vi "Unflatten JSONpath Array to Object.vi"(8 "error in (no error)":errorcluster, 9 "JSON Items":string[](array[string]), 11 "$Paths":string[](array[string])) -> (0 "error out":errorcluster, 3 "<JSON>":string)   [LabVIEW 2017, in "JSONtext.lvlib"]
doc: "Takes arrays of $Paths items and generates a Object containing those $Paths. Does not support multi-point paths.\n\nFor example: the $Paths (Items):\n$.A.B1 (1)\n$.A.B2 (\"x\")\n$.A2 (true)\n$.A3.C (123)\nproduce the JSON: {\"A\":{\"B1\":1\"B2:\"x\"},\"A2\":true,\"A3\":{\"C\":123}}"
uses:
  JSONtext.lvlib
  Parsing/Replace at Offset.vi
  support/Trim Input JSON (and null).vi
  Parsing/Advance past whitespace.vi
  <vilib>/JDP Science/JDP Science Common Utilities/Trim Whitespace__JDP.vi
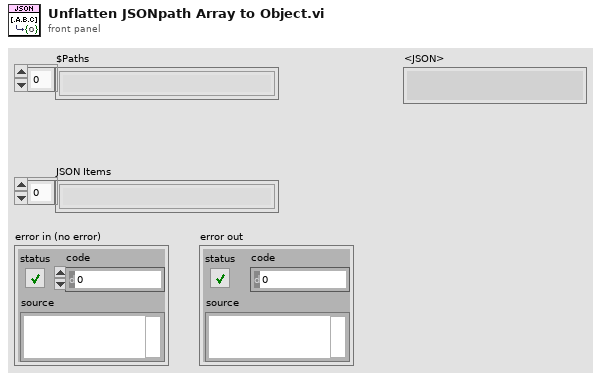
[diagram p1: front panel]
types:
  T1 = typedef "JSONtext.lvlib/Found Items.ctl" = cluster{"Item offset":i32, "Offset past Item":i32, "Name offset":i32, "Offset past Name":i32, "Found":bool, "Item Type":T2, "Item Index":i32}
  T2 = typedef "JSONtext.lvlib/Parsing State.ctl" = enum16{"Parser Error", "Object", "Array", "String", "Number/Other", "Leading Whitespace", "Object end", "Array end", "Value end"}
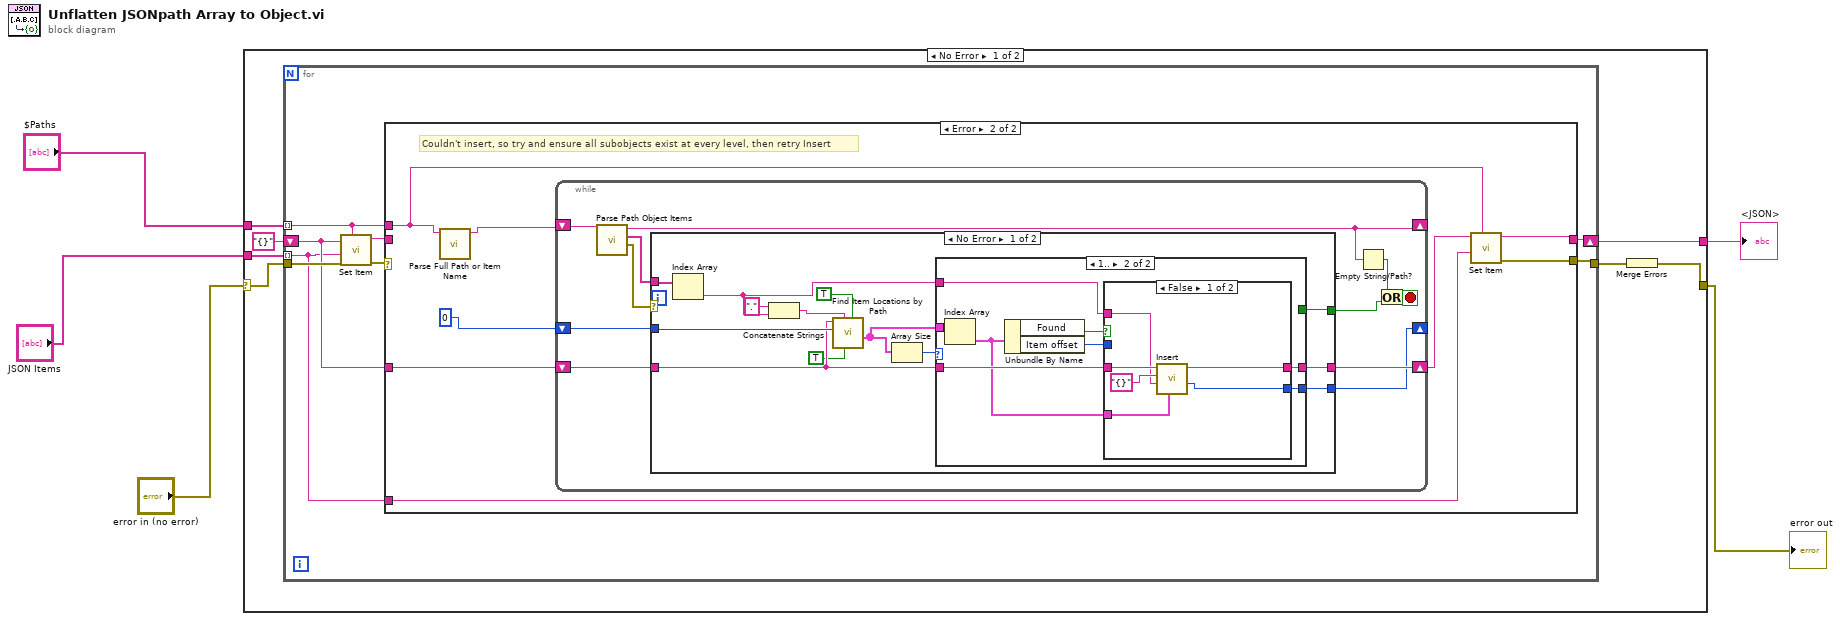
[diagram p0: block diagram]
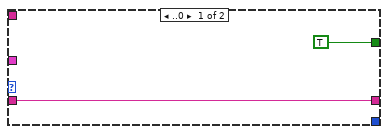
[diagram p3: hidden frame]
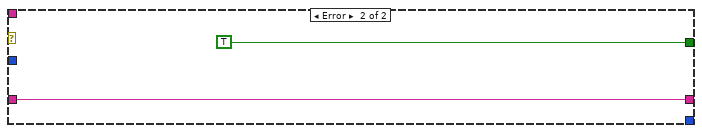
[diagram p5: hidden frame]
diagram:
  n1 = case shown="No Error" "error in (no error)" {
    selector: "error in (no error)" -> [w9 w75]
    tunnel: "$Paths" -> [w12 _]
    tunnel: "JSON Items" -> [w10 _]
    tunnel: [w8 _] -> w4
    tunnel: [w6 w75] -> w5
    frame No Error {
      n2 = for {
        tunnel: w12 -> [w18] mode=indexing
        shift-right: [w15] -> w8
        shift-left: "{}" ("<JSON>") -> [w17]
        tunnel: w10 -> [w13] mode=indexing
        tunnel: w9 -> [w20]
        tunnel: [w14] -> w7
        n3 = call "Set Item.vi"("$Path or Item Name"=w18, "error in (no error)"=w20, "JSON to Insert"=w13, "JSON"=w17) -> ("error out"=w19:errorcluster, "<JSON>"=w16:string)  [unwired: 4 in, 1 out]
        n4 = case shown="Error" w19 {
          selector: w19 -> [w21 _]
          tunnel: w18 -> [_ w25]
          tunnel: w17 -> [_ w30]
          tunnel: w16 -> [w22 _]
          tunnel: [w22 w28] -> w15
          tunnel: [w21 w27] -> w14
          tunnel: w13 -> [_ w26]
          frame No Error {
          }
          frame Error {
            # "Couldn't insert, so try and ensure all subobjects exist at every level, then retry Insert"
            n5 = call "Parse Full Path or Item Name.vi"("Full Path (with $) or Name"=w25) -> ("Relative Path or JSON-format name"=w23:string)  [unwired: 10 in]
            n6 = while {
              shift-right: [w39] -> _
              shift-left: w23 -> [w33]
              shift-right: [w36] -> w29
              shift-left: w30 -> [w37]
              shift-right: [w31] -> _
              shift-left: 0 ("Offset") -> [w32]
              stop <- w35 stop-if-true
              n7 = call "Parse Path Object Items.vi"("Path with leading Object element"=w33) -> ("error out"=w40:errorcluster, "<JSON>items names"=w38:string[], "Rest or Path"=w39:string)  [unwired: 8 in]
              n8 = case shown="No Error" w40 {
                tunnel: w38 -> [w54 _]
                tunnel: w37 -> [w51 w73]
                tunnel: [w53 w73] -> w36
                tunnel: [w43 TRUE] -> w34
                tunnel: w32 -> [w52 _]
                tunnel: [w48 _] -> w31
                frame No Error {
                  n9 = Index Array(array=w54) -> (element=w46:string)  [unwired: 1 in]
                  n10 = Concatenate Strings("." ("string"), w46) -> (w47:string)
                  n11 = call "Find Item Locations by Path.vi"("Insertion point if not found"=TRUE, "Only return first found"=TRUE, "Path"=w47, "Offset"=w52, "JSON"=w51) -> ("Items"=w45:T1[])  [unwired: 5 in, 1 out]
                  n12 = Array Size(array=w45) -> (size(s)=w44:i32)
                  n13 = case shown="1.." w44 {
                    tunnel: [w56 w64] -> w53
                    tunnel: w51 -> [w56 w63]
                    tunnel: [_ w60] -> w48
                    tunnel: w46 -> [_ w58]
                    tunnel: w45 -> [_ w57]
                    tunnel: [TRUE _] -> w43
                    frame ..0 {
                    }
                    frame 1.. {
                      n14 = Index Array(array=w57) -> (element=w61:T1)  [unwired: 1 in]
                      n15 = Unbundle By Name(w61) -> ("Found"=w62:bool, "Item offset"=w59:i32)
                      n16 = case shown="False" w62 {
                        tunnel: [w68 w72] -> w64
                        tunnel: w63 -> [w69 w72]
                        tunnel: w61 -> [w70 _]
                        tunnel: w58 -> [w66 _]
                        tunnel: [w65 w71] -> w60
                        tunnel: w59 -> [_ w71]
                        frame False {
                          n17 = call "Insert.vi"("Item"=w70, "<JSON>name"=w66, "JSON to Insert"="{}", "JSON in"=w69) -> ("Inserted Item Offset"=w65:i32, "string"=w68:string)  [unwired: 5 in, 1 out]
                        }
                        frame True {
                        }
                      }
                    }
                  }
                }
                frame Error {
                }
              }
              n18 = Empty String/Path?(string/path=w39) -> (empty?=w41:bool)
              n19 = Or(x=w41, y=w34) -> (x .or. y?=w35:bool)
            }
            n20 = call "Set Item.vi"("$Path or Item Name"=w25, "JSON to Insert"=w26, "JSON"=w29) -> ("error out"=w27:errorcluster, "<JSON>"=w28:string)  [unwired: 5 in, 1 out]
          }
        }
      }
      n21 = Merge Errors(w7) -> (w6:errorcluster)
    }
    frame Error {
    }
  }
  "error out" <- w5
  "<JSON>" <- w4
